vi "PopulateParameterHyperCube-FromList.vi"(8 "error in (no error)":errorcluster, 11 "Range and Resolution Preview":T1(array[cluster])) -> (0 "error out":errorcluster, 2 "2D Array":dbl[][](array[numeric]), 3 "Parameter Sequence":cluster{dbl[]}[](array[cluster]))   [LabVIEW 2019]
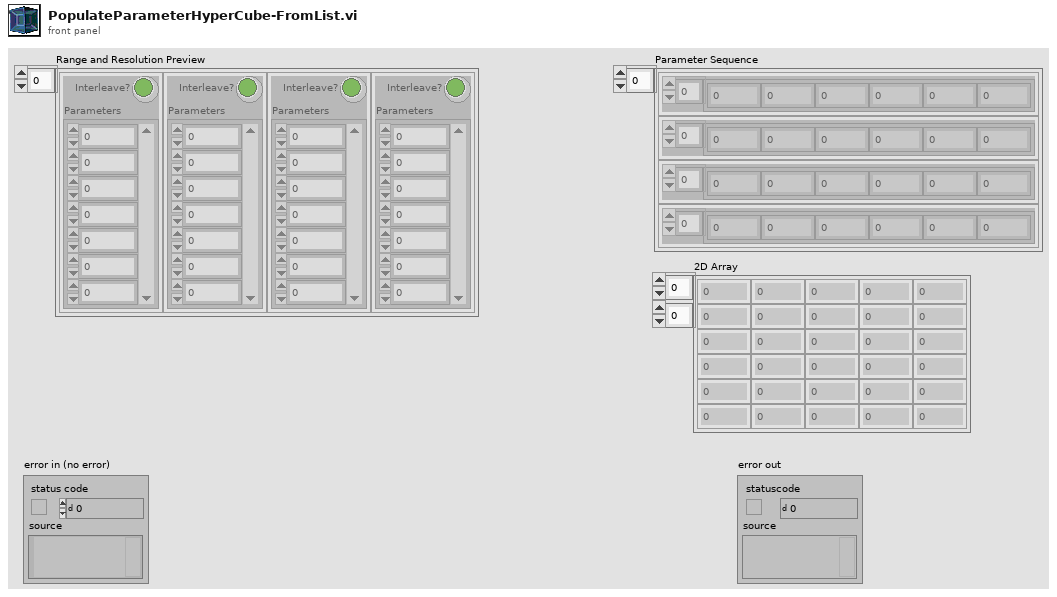
[diagram p1: front panel]
types:
  T1 = cluster{"Parameters":dbl[], "Interleave?":bool}[]
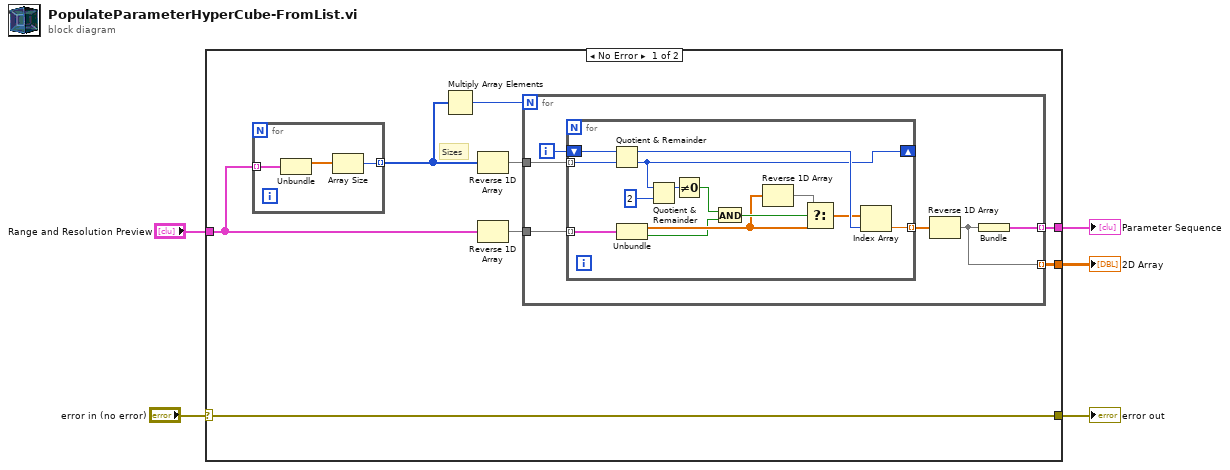
[diagram p0: block diagram]
diagram:
  n1 = case shown="No Error" "error in (no error)" {
    selector: "error in (no error)" -> [w9 w37]
    tunnel: [w12 _] -> w5
    tunnel: [w9 w37] -> w3
    tunnel: [w8 _] -> w2
    tunnel: "Range and Resolution Preview" -> [w7 _]
    frame No Error {
      # "Sizes"
      n2 = for {
        tunnel: w7 -> [w16] mode=indexing
        tunnel: [w14] -> w6 mode=indexing
        n3 = Unbundle(w16) -> ("Parameters"=w15:dbl[])  [unwired: 1 out]
        n4 = Array Size(array=w15) -> (size(s)=w14:i32)
      }
      n5 = Multiply Array Elements(1:w6) -> (0:w13:i32)
      n6 = Reverse 1D Array(array=w6) -> (reversed array=w11:i32[])
      n7 = Reverse 1D Array(array=w7) -> (reversed array=w10:T1)
      n8 = for {
        N: w13 -> [_]
        tunnel: w10 -> [w18]
        tunnel: w11 -> [w19]
        tunnel: [w20] -> w12 mode=indexing
        tunnel: [w17] -> w8 mode=indexing
        i -> [w22]
        n9 = for {
          tunnel: w19 -> [w36] mode=indexing
          shift-right: [w31] -> _
          shift-left: w22 -> [w35]
          tunnel: w18 -> [w34] mode=indexing
          tunnel: [w32] -> w21 mode=indexing
          n10 = Quotient & Remainder(x=w35, y=w36) -> (x-y*floor(x/y)=w33:i32, floor(x/y)=w31:i32)
          n11 = Unbundle(w34) -> ("Parameters"=w24:dbl[], "Interleave?"=w23:bool)
          n12 = Quotient & Remainder(x=w31, y=2) -> (x-y*floor(x/y)=w29:i32)  [unwired: 1 out]
          n13 = Not Equal To 0?(x=w29) -> (x != 0?=w28:bool)
          n14 = And(x=w28, y=w23) -> (x .and. y?=w27:bool)
          n15 = Reverse 1D Array(array=w24) -> (reversed array=w26:dbl[])
          n16 = Select(t=w26, s=w27, f=w24) -> (s? t:f=w25:dbl[])
          n17 = Index Array(array=w25, index=w33) -> (element=w32:dbl)
        }
        n18 = Reverse 1D Array(array=w21) -> (reversed array=w17:dbl[])
        n19 = Bundle(w17) -> (w20:cluster{dbl[]})  [unwired: 1 in]
      }
    }
    frame Error {
    }
  }
  "Parameter Sequence" <- w5
  "error out" <- w3
  "2D Array" <- w2
